vi "Do.vi"(8 "error in (no error)":errorcluster, 10 "Actor in":refnum<class "Actor.lvclass">, 11 "Update Display Msg":refnum<class "Update Display Msg.lvclass">) -> (0 "error out":errorcluster, 2 "Actor out":refnum<class "Actor.lvclass">)   [LabVIEW 2017, in "Simulated Screen Interface.lvlib" / "Update Display Msg.lvclass"]
doc: "This VI delivers the message to the actor by calling the appropriate method(s) on the actor."
uses:
  Update Display Msg.lvclass
  C:/Users/chris/Documents/GitHub/Tetris/RT Code/Screen Interface/Screen Interface Messages/Display Game Board Msg/Display Game Board Msg.lvclass
  <vilib>/ActorFramework/Actor/Actor.lvclass
  Simulated Screen Interface/Simulated Screen Interface.lvclass
  C:/Program Files (x86)/National Instruments/LabVIEW 2017/vi.lib/ActorFramework/Actor/Actor.lvclass
  Screen Interface/Screen Interface Messages/Display Game Board Msg/Display Game Board Msg.lvclass/Display Game Board Msg.ctl
  Screen Interface/Screen Interface Messages/Display Game Board Msg/Display Game Board Msg.lvclass
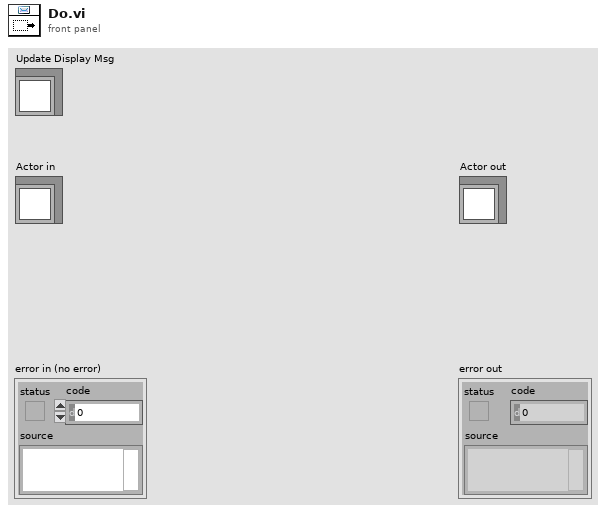
[diagram p1: front panel]
types:
  T1 = cluster{"Board State":u32[][], "Active Pixels":cluster{"Column":u8, "Row":u8, "Color":u32}[]}
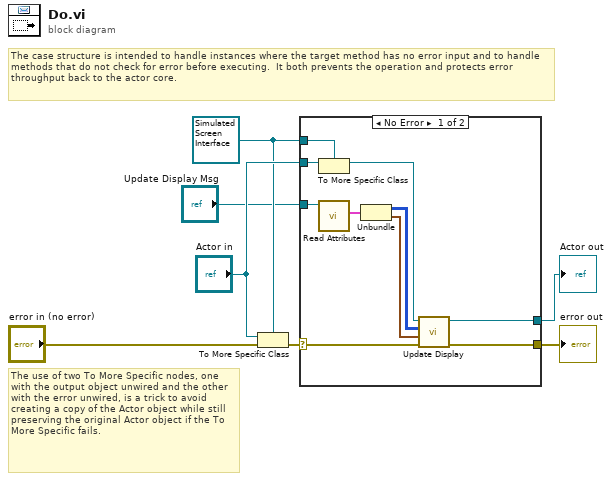
[diagram p0: block diagram]
diagram:
  w2 = refnum<class "Simulated Screen Interface.lvclass"> refnum ("Actor in")
  # "The use of two To More Specific nodes, one with the output object unwired and the other with the error unwired, is a trick to avoid creating a copy of the Actor object while still preserving the original Actor object if the To More Specific fails."
  # "The case structure is intended to handle instances where the target method has no error input and to handle methods that do not check for error before executing.  It both prevents the operation and protects error throughput back to the actor core."
  n1 = To More Specific Class(target class=w2, reference="Actor in", error in="error in (no error)") -> (error out=w6:errorcluster)  [unwired: 1 out]
  n2 = case shown="No Error" w6 {
    selector: w6 -> [w15 w19]
    tunnel: [w17 w19] -> w5
    tunnel: [w16 w18] -> w4
    tunnel: "Actor in" -> [w14 w18]
    tunnel: w2 -> [w13 _]
    tunnel: "Update Display Msg" -> [w10 _]
    frame No Error {
      n3 = To More Specific Class(target class=w13, reference=w14) -> (specific class reference=w12:refnum<class "Simulated Screen Interface.lvclass">)  [unwired: 1 in, 1 out]
      n4 = call "Read Attributes.vi"("Display Game Board Msg"=w10) -> ("Payload"=w11:T1)  [unwired: 10 in]
      n5 = Unbundle(w11) -> ("Board State"=w9:u32[][], "Active Pixels"=w8:cluster{"Column":u8, "Row":u8, "Color":u32}[])
      n6 = call-dynamic "Update Display.vi"("error in (no error)"=w15, "Active Pixels"=w8, "Board State"=w9, "Simulated Screen Interface in"=w12) -> ("error out"=w17:errorcluster, "Simulated Screen Interface out"=w16:refnum<class "Simulated Screen Interface.lvclass">)  [unwired: 6 in]
    }
    frame Error {
      # "If type check fails, pass the original object out again."
    }
  }
  "error out" <- w5
  "Actor out" <- w4
